vi "TP_TimeLeftUntilPosition.vi"(8 "error in (no error)":errorcluster, 11 "TrapezoidalProfile in":refnum<class "TrapezoidalProfile.lvclass">) -> (0 "error out":errorcluster, 3 "TrapezoidalProfile out":refnum<class "TrapezoidalProfile.lvclass">)   [LabVIEW 2018, in "TrapezoidalProfile.lvclass"]
uses:
  TrapezoidalProfile.lvclass
  TrapezoidalProfile.lvclass/TrapezoidalProfile.ctl
panel:
  out "Time Left Until":dbl
  in  "Position":dbl
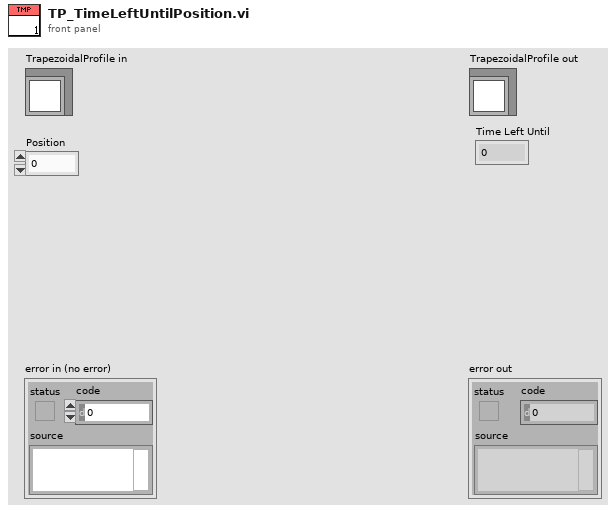
[diagram p1: front panel]
types:
  T1 = typedef "TrapezoidalProfile.lvclass/State.ctl" = cluster{"Position (u)":dbl, "Velocity (u/s)":dbl}
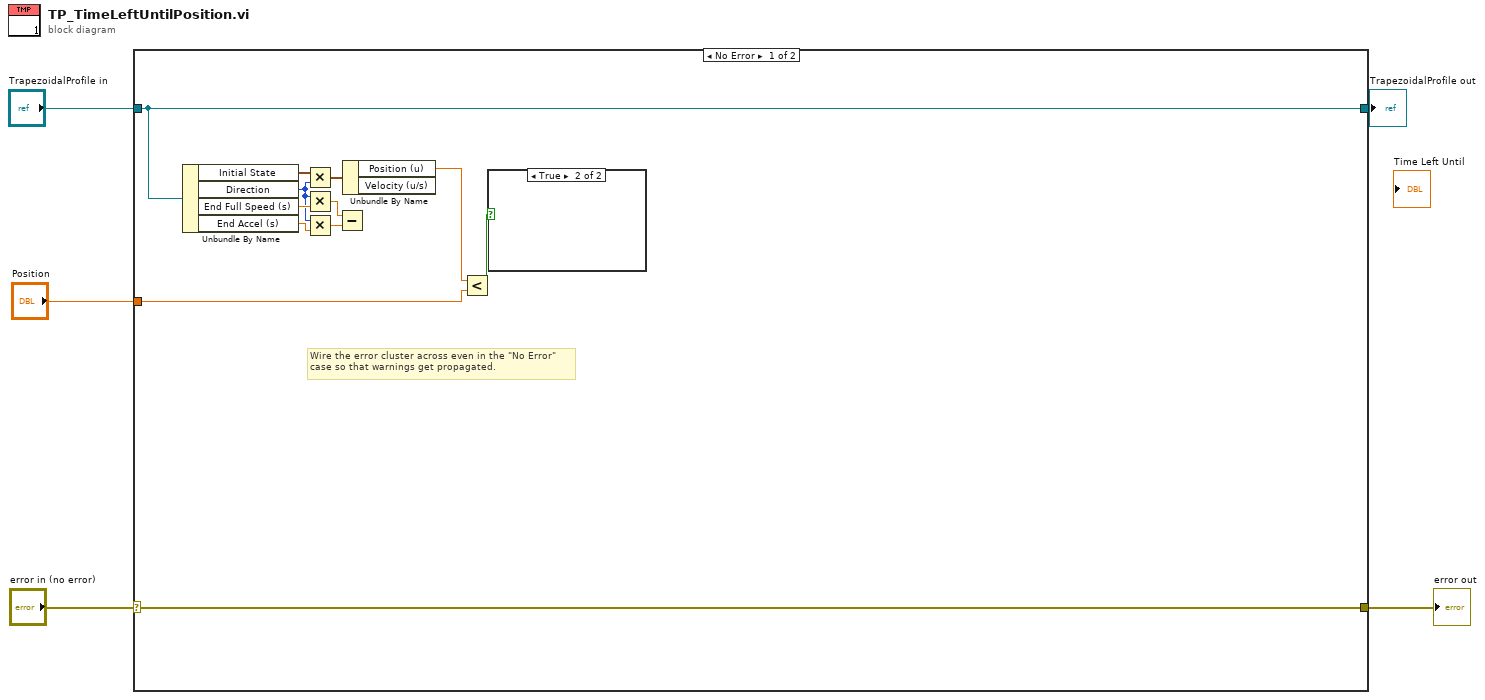
[diagram p0: block diagram]
diagram:
  n1 = case shown="No Error" "error in (no error)" {
    selector: "error in (no error)" -> [w17 w19]
    tunnel: [w17 w19] -> w4
    tunnel: [w16 w18] -> w2
    tunnel: "TrapezoidalProfile in" -> [w16 w18]
    tunnel: "Position" -> [w6 _]
    frame No Error {
      # "Wire the error cluster across even in the \"No Error\"\ncase so that warnings get propagated."
      n2 = Unbundle By Name(w16) -> ("Initial State"=w15:T1, "Direction"=w12:i32, "End Full Speed (s)"=w13:dbl, "End Accel (s)"=w11:dbl)
      n3 = Multiply(x=w15, y=w12) -> (x*y=w14:T1)
      n4 = Multiply(x=w12, y=w13) -> (x*y=w10:dbl)
      n5 = Multiply(x=w12, y=w11) -> (x*y=w9:dbl)
      n6 = Subtract(x=w10, y=w9) -> ()  [unwired: 1 out]
      n7 = Unbundle By Name(w14) -> ("Position (u)"=w7:dbl)  [unwired: 1 out]
      n8 = Less?(x=w7, y=w6) -> (x < y?=w8:bool)
      n9 = case shown="True" w8 {
        frame False {
        }
        frame True {
        }
      }
    }
    frame Error {
    }
  }
  "error out" <- w4
  "TrapezoidalProfile out" <- w2
